vi "Word Get ActiveX References.vi"(0 "report in":refnum<class "NI_report.lvclass">, 11 "error in (no error)":errorcluster) -> (3 "Word._Application":refnum<k7>, 4 "report out":refnum<class "NI_report.lvclass">, 6 "Word.Documents":refnum<k7>, 8 "Word._Document":refnum<k7>, 10 "Word.Tables":refnum<k7>, 14 "Word.InlineShapes":refnum<k7>, 15 "error out":errorcluster)   [LabVIEW 2020, in "NI_Word.lvclass"]
doc: "Returns ActiveX references to Microsoft Word."
uses:
  <vilib>/Utility/NIReport.llb/Word/NI_Word.lvclass
  <vilib>/Utility/NIReport.llb/NI_report.lvclass
  C:/Program Files (x86)/National Instruments/LabVIEW 2020/vi.lib/Utility/NIReport.llb/NI_report.lvclass
  <vilib>/Utility/NIReport.llb/Word/NI_Word.lvclass/NI_Word.ctl
  <vilib>/Utility/NIReport.llb/NI_ReportGenerationCore.lvlib
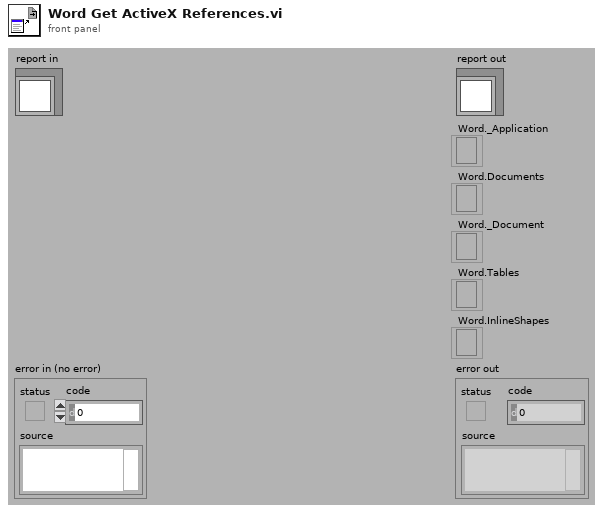
[diagram p1: front panel]
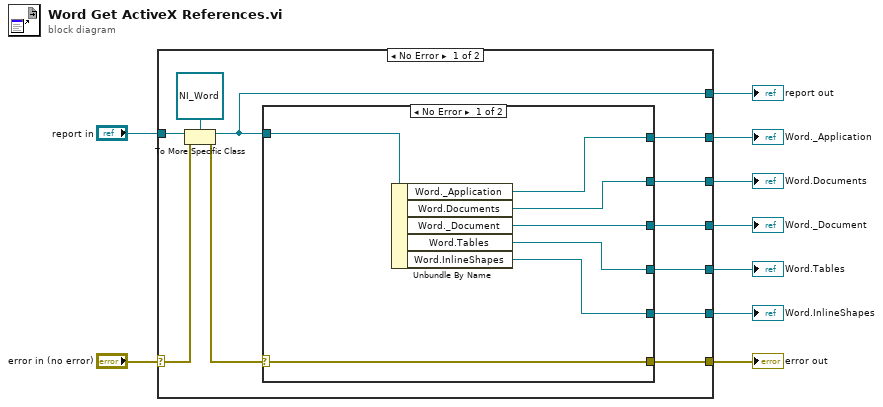
[diagram p0: block diagram]
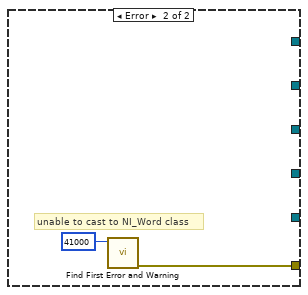
[diagram p2: hidden frame]
diagram:
  n1 = case shown="No Error" "error in (no error)" {
    selector: "error in (no error)" -> [w15 w31]
    tunnel: [w20 w31] -> w8
    tunnel: [w17 w30] -> w6
    tunnel: "report in" -> [w18 w30]
    tunnel: [w14 _] -> w5
    tunnel: [w13 _] -> w4
    tunnel: [w12 _] -> w3
    tunnel: [w11 _] -> w2
    tunnel: [w10 _] -> w1
    frame No Error {
      n2 = To More Specific Class(target class=refnum<class "NI_Word.lvclass"> refnum ("report in"), reference=w18, error in=w15) -> (specific class reference=w17:refnum<class "NI_Word.lvclass">, error out=w16:errorcluster)
      n3 = case shown="No Error" w16 {
        selector: w16 -> [w26 _]
        tunnel: [w26 w28] -> w20
        tunnel: w17 -> [w27 _]
        tunnel: [w25 _] -> w14
        tunnel: [w24 _] -> w13
        tunnel: [w23 _] -> w12
        tunnel: [w22 _] -> w11
        tunnel: [w21 _] -> w10
        frame No Error {
          n4 = Unbundle By Name(w27) -> ("Word._Application"=w24:refnum<k7>, "Word.Documents"=w23:refnum<k7>, "Word._Document"=w25:refnum<k7>, "Word.Tables"=w21:refnum<k7>, "Word.InlineShapes"=w22:refnum<k7>)
        }
        frame Error {
          # "unable to cast to NI_Word class"
          n5 = call <vilib>:"Find First Error and Warning.vi"("error code"=41000) -> ("error out"=w28:errorcluster)  [unwired: 2 in, 4 out]
        }
      }
    }
    frame Error {
    }
  }
  "error out" <- w8
  "report out" <- w6
  "Word._Application" <- w4
  "Word.Documents" <- w3
  "Word._Document" <- w5
  "Word.Tables" <- w1
  "Word.InlineShapes" <- w2
